vi "data_mapper.vi"(11 "input":T2(array[cluster])) -> (3 "output":T1(array[cluster]))   [LabVIEW 2021]
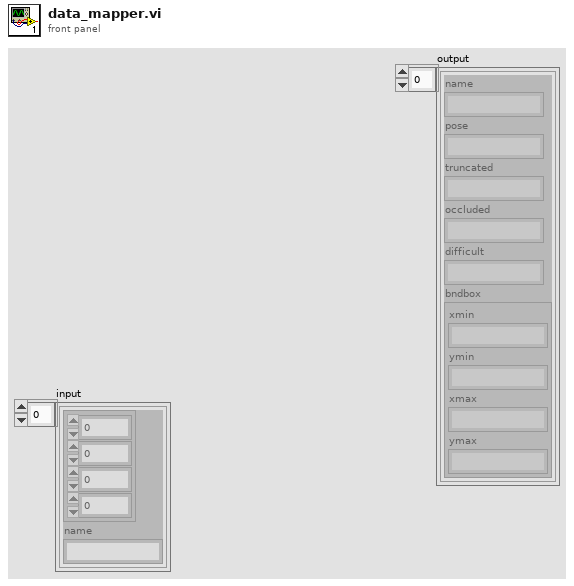
[diagram p1: front panel]
types:
  T1 = cluster{"name":string, "pose":string, "truncated":string, "occluded":string, "difficult":string, "bndbox":cluster{"xmin":string, "ymin":string, "xmax ":string, "ymax":string}}[]
  T2 = cluster{cluster{i32, i32, i32, i32}, "name":string}[]
  T3 = cluster{"name":string, "pose":string, "truncated":string, "occluded":string, "difficult":string, "bndbox":cluster{"xmin":string, "ymin":string, "xmax ":string, "ymax":string}}
  T4 = cluster{"xmin":string, "ymin":string, "xmax ":string, "ymax":string}
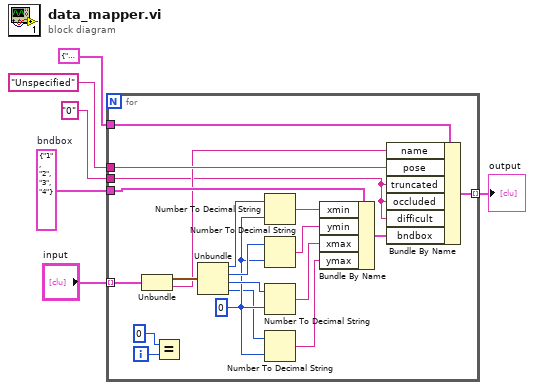
[diagram p0: block diagram]
diagram:
  w5 = T4 {"xmin"="1", "ymin"="2", "xmax "="3", "ymax"="4"}  # bndbox
  n1 = for {
    tunnel: "input" -> [w26] mode=indexing
    tunnel: T3 {"name"="", "pose"="Unspecified", "truncated"="0", "occluded"="0", "difficult"="0", "bndbox"={"xmin"="", "ymin"="", "xmax "="", "ymax"=""}} ("object") -> [w24]
    tunnel: w5 -> [w23]
    tunnel: "0" ("name") -> [w7]
    tunnel: "Unspecified" ("pose") -> [w22]
    tunnel: [w10] -> w1 mode=indexing
    i -> [w11]
    w17 = i16 0 ("width (-)")
    n2 = Unbundle(w26) -> (w25:cluster{i32, i32, i32, i32}, "name"=w9:string)
    n3 = Equal?(x=0, y=w11) -> ()  [unwired: 1 out]
    n4 = Unbundle(w25) -> (w21:i32, w19:i32, w18:i32, w16:i32)
    n5 = Number To Decimal String(number=w21, width (-)=w17) -> (decimal integer string=w20:string)
    n6 = Number To Decimal String(number=w19, width (-)=w17) -> (decimal integer string=w15:string)
    n7 = Number To Decimal String(number=w18, width (-)=w17) -> (decimal integer string=w14:string)
    n8 = Number To Decimal String(number=w16, width (-)=w17) -> (decimal integer string=w13:string)
    n9 = Bundle By Name(cluster=w23, "xmin"=w20, "ymin"=w15, "xmax"=w14, "ymax"=w13) -> (w8:T4)
    n10 = Bundle By Name(cluster=w24, "name"=w9, "pose"=w22, "truncated"=w7, "occluded"=w7, "difficult"=w7, "bndbox"=w8) -> (w10:T3)
  }
  "output" <- w1
